vi "(SubVI) Calc_number_of_digits.vi"(3 "target_digit":dbl, 4 "Input_2":dbl, 5 "Input_1":dbl) -> (0 "output_digit":dbl, 1 "remain_2":dbl, 2 "remain_1":dbl)   [LabVIEW 2018]
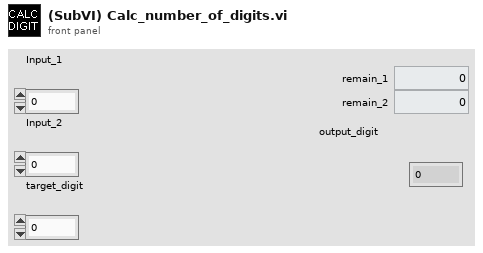
[diagram p1: front panel]
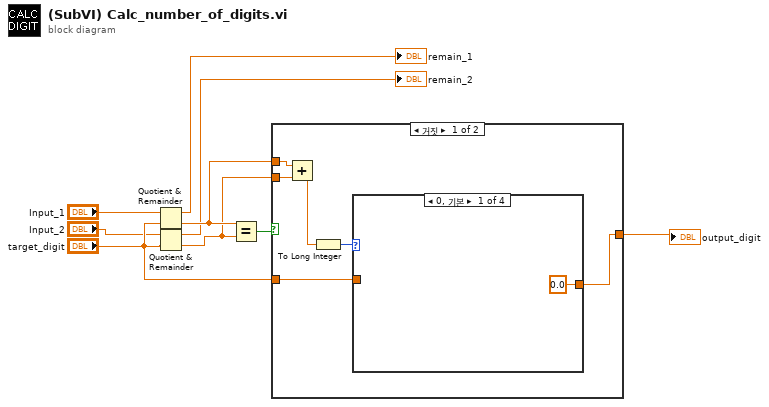
[diagram p0: block diagram]
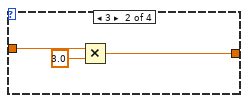
[diagram p2: hidden frame]
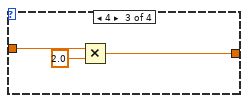
[diagram p3: hidden frame]
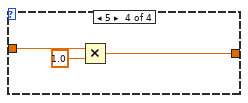
[diagram p4: hidden frame]
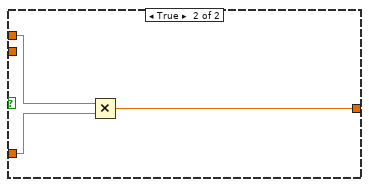
[diagram p5: hidden frame]
diagram:
  n1 = Quotient & Remainder(x="Input_1", y="target_digit") -> (x-y*floor(x/y)=→"remain_1":dbl, floor(x/y)=w4:dbl)
  n2 = Quotient & Remainder(x="Input_2", y="target_digit") -> (x-y*floor(x/y)=→"remain_2":dbl, floor(x/y)=w3:dbl)
  n3 = Equal?(x=w4, y=w3) -> (x = y?=w9:bool)
  n4 = case shown="거짓" w9 {
    tunnel: w4 -> [w15 w28]
    tunnel: "target_digit" -> [w11 w27]
    tunnel: [w10 w26] -> w6
    tunnel: w3 -> [w14 _]
    frame False {
      n5 = Add(x=w15, y=w14) -> (x+y=w12:dbl)
      n6 = To Long Integer(number=w12) -> (32bit integer=w13:i32)
      n7 = case shown="0, 기본" w13 {
        tunnel: w11 -> [_ w19 w22 w25]
        tunnel: [0.0 w17 w20 w23] -> w10
        frame 0, Default {
        }
        frame 3 {
          n8 = Multiply(x=w19, y=3.0) -> (x*y=w17:dbl)
        }
        frame 4 {
          n9 = Multiply(x=w22, y=2.0) -> (x*y=w20:dbl)
        }
        frame 5 {
          n10 = Multiply(x=w25, y=1.0) -> (x*y=w23:dbl)
        }
      }
    }
    frame True {
      n11 = Multiply(x=w28, y=w27) -> (x*y=w26:dbl)
    }
  }
  "output_digit" <- w6
